vi "DriveFineAjust.vi"(8 "Fine Ajust F/B":dbl, 9 "Fine Ajust L/R":dbl, 10 "Right Side Normal":dbl, 11 "Left Side Normal":dbl) -> ()   [LabVIEW 2012]
uses:
  <vilib>/Rock Robotics/WPI/RobotDrive/WPI_RobotDriveGetSetRefNum.vi
  <vilib>/Rock Robotics/WPI/RobotDrive/WPI_RobotDriveArcadeDrive_Standard(NoSaturation).vi
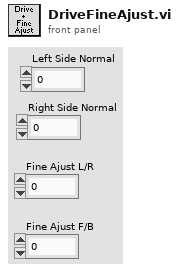
[diagram p1: front panel]
types:
  T1 = typedef "WPI_RobotDriveDevRef.ctl" = cluster{"DevStatus":errorcluster, "Motors[]":T2[], "Square Inputs":bool, "Max Output":dbl, "Isochronous":bool}
  T2 = typedef "WPI_MotorControlDeviceRef.ctl" = cluster{"DeviceStatus":errorcluster, "Type":enum16{"PWM", "CAN"}, "PWM":cluster{"Digital Module":T3, "PWM Channel":T4, "DeadBand":T5}, "CAN":cluster{"Device Number":u8, "Control Mode":T6, "Semaphore":T7, "Max Vout":dbl}, "Invert":bool, "TransformRef":T8, "InvTransformRef":T8}
  T3 = typedef "FPGA_TypedefDigitalModule.ctl" = enum16{"Digital Module 1", "Digital Module 2"}
  T4 = typedef "FPGA_DIOPWMChannel.ctl" = enum8{"PWM 1", "PWM 2", "PWM 3", "PWM 4", "PWM 5", "PWM 6", "PWM 7", "PWM 8", "PWM 9", "PWM 10", "Invalid"}
  T5 = typedef "WPI_PWMDeadband.ctl" = cluster{"Name":string, "maxPositivePwm":i32, "minPositivePwm":i32, "centerPwm":i32, "maxNegativePwm":i32, "minNegativePwm":i32, "angularRange":u16}
  T6 = typedef "WPI_CANJaguar_ControlMode.ctl" = enum8{"Percent VBus", "Current", "Speed", "Position", "Voltage"}
  T7 = typedef "Semaphore RefNum" = refnum<k1>
  T8 = typedef "WPI_PWMTransform_ConPane.ctl" = refnum<vi>
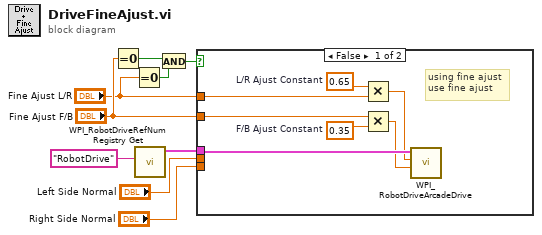
[diagram p0: block diagram]
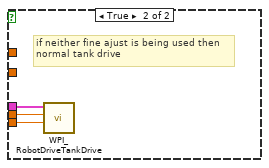
[diagram p2: hidden frame]
diagram:
  n1 = Equal To 0?(x="Fine Ajust F/B") -> (x = 0?=w1:bool)
  n2 = Equal To 0?(x="Fine Ajust L/R") -> (x = 0?=w2:bool)
  n3 = call <vilib>:"WPI_RobotDriveRefNum Registry Get.vi"("refnum name"="RobotDrive") -> ("RobotDriveDevRef"=w7:T1)  [unwired: 1 in, 9 out]
  n4 = And(x=w1, y=w2) -> (x .and. y?=w3:bool)
  n5 = case shown="False" w3 {
    tunnel: "Right Side Normal" -> [_ w19]
    tunnel: "Left Side Normal" -> [_ w18]
    tunnel: w7 -> [w16 w17]
    tunnel: "Fine Ajust L/R" -> [w13 _]
    tunnel: "Fine Ajust F/B" -> [w11 _]
    frame False {
      w12 = 0.35  # F/B Ajust Constant
      w15 = 0.65  # L/R Ajust Constant
      # "using fine ajust\nuse fine ajust"
      n6 = Multiply(x=w15, y=w13) -> (x*y=w14:dbl)
      n7 = Multiply(x=w11, y=w12) -> (x*y=w10:dbl)
      n8 = call-poly <vilib>:"WPI_RobotDriveArcadeDrive.vi"("Y axis value"=w10, "X axis value"=w14, "RobotDriveDevRef"=w16) -> ()  [unwired: 6 in, 3 out]
    }
    frame True {
      # "if neither fine ajust is being used then\nnormal tank drive"
      n9 = call <vilib>:"WPI_RobotDriveTankDrive.vi"("Right axis value"=w19, "Left axis value"=w18, "RobotDriveDevRef"=w17) -> ()  [unwired: 6 in, 3 out]
    }
  }
